vi "Create Internal Error Enqueuer.vi"(8 "error in (no error)":errorcluster) -> (0 "error out":errorcluster, 2 "Error Enqueuer":refnum<user-event>, 3 "Internal-Error":refnum<event-registration>)   [LabVIEW 2018, in "Scripting.lvlib" / "Actor.lvclass"]
uses:
  Actor.lvclass
  Internal-Error.ctl
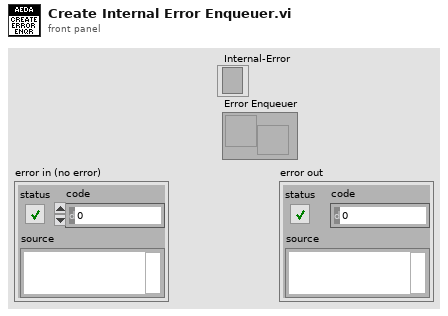
[diagram p1: front panel]
types:
  T1 = typedef "Scripting.lvlib/Actor.lvclass/Internal-Error.ctl" = cluster{"Error":errorcluster}
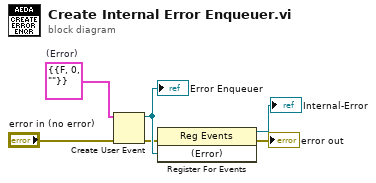
[diagram p0: block diagram]
diagram:
  w5 = T1 {"Error"={"status"=FALSE, "code"=0, "source"=""}}  # (Error)
  n1 = Create User Event(user event datatype=w5, error in="error in (no error)") -> (user event=w4:refnum<user-event>, error out=w3:errorcluster)
  "Error Enqueuer" <- w4
  n2 = register-events(error in=w3, w4) -> (reference out=→"Internal-Error":refnum<event-registration>, error out=→"error out":errorcluster)  [unwired: 1 in]
